vi "Core Action.vi"(8 "error in (no error)":errorcluster, 10 "SECS-II Class":refnum<class "SECS-II Class.lvclass">, 11 "30-Host Requests Equipment to Set Time in":refnum<class "30-Host Requests Equipment to Set Time.lvclass">) -> (0 "error out":errorcluster, 2 "SECS-II Class Out":refnum<class "SECS-II Class.lvclass">, 3 "30-Host Requests Equipment to Set Time out":refnum<class "30-Host Requests Equipment to Set Time.lvclass">)   [LabVIEW 2020, in "SECS Scenarios.lvlib" / "30-Host Requests Equipment to Set Time.lvclass"]
uses:
  30-Host Requests Equipment to Set Time.lvclass
  D:/Dropbox/SECS/SECS_GEM v1.1.0/Com/SECS Scenarios/Scenarios Class/Scenarios Class.lvclass
  SECS Communication/SECS-II Class/SECS-II Class.lvclass
  SECS Communication/S2 Message Class/S2 Message Class.lvclass
  D:/Dropbox/SECS/SECS_GEM v1.1.0/Com/SECS Communication/SECS-II Class/SECS-II Class.lvclass
  Scenarios Class/Reply State.ctl
  Scenarios Class/Scenarios Class.lvclass/Scenarios Class.ctl
  Scenarios Class/Write Reply State.vi
  Scenarios Class/Read HSMS Class.vi
  SECS Communication/HSMS Class/HSMS Class.lvclass
  Scenarios Class/Scenarios Class.lvclass
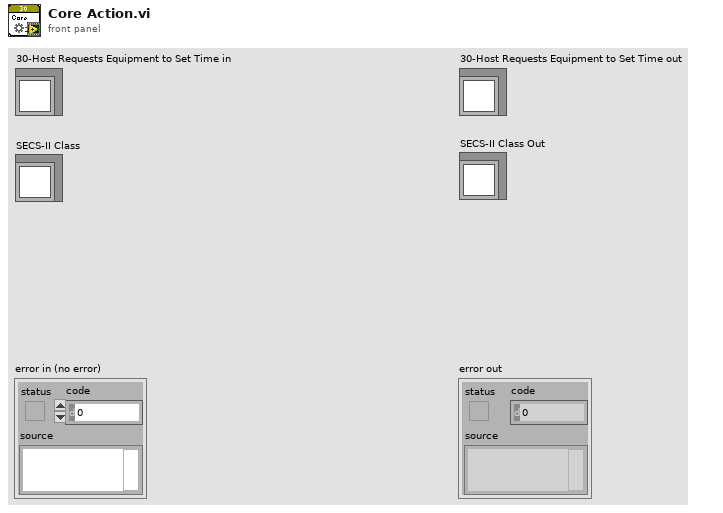
[diagram p1: front panel]
types:
  T1 = typedef "SECS Scenarios.lvlib/Scenarios Class.lvclass/Reply State.ctl" = enum16{"OK", "Illegal Data", "Unknown Stream", "Unknown Function", "Off-Line", "T3 Timeout", "Inner-Timeout"}
  T2 = typedef "SECS Communication.lvlib/S2 Message Class.lvclass/S2F32.ctl" = enum16{"ok", "not done"}
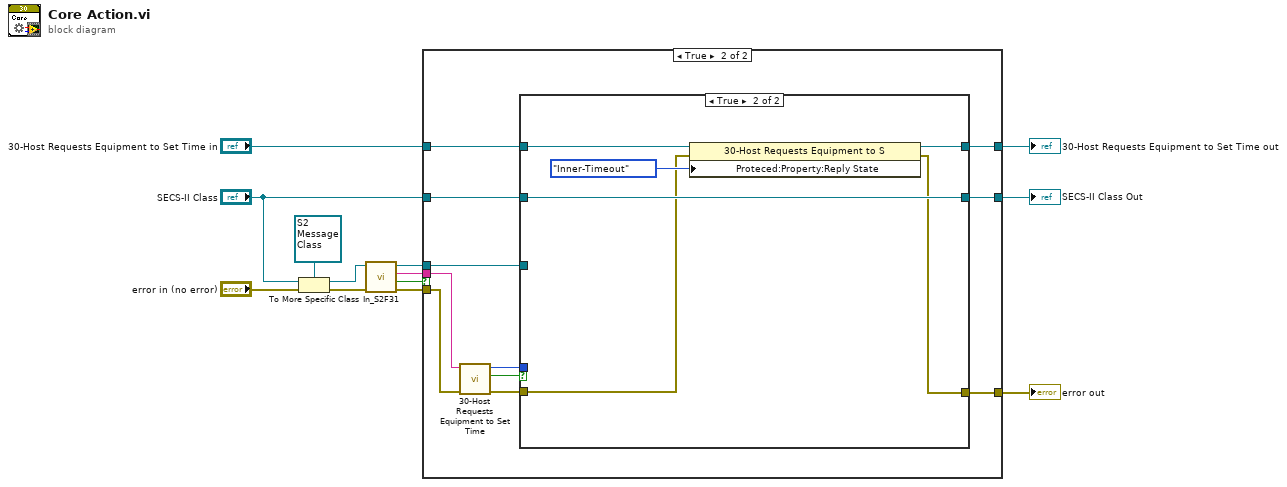
[diagram p0: block diagram]
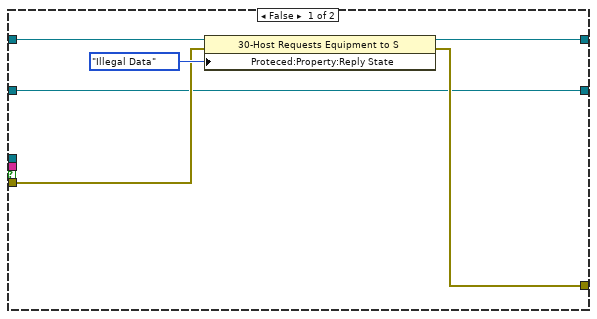
[diagram p2: hidden frame]
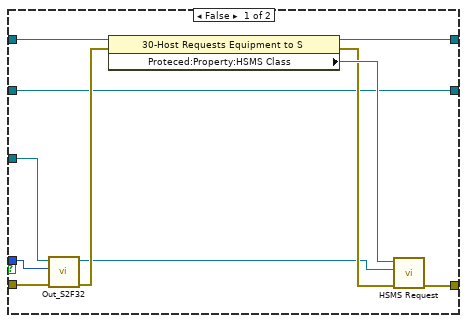
[diagram p3: hidden frame]
diagram:
  n1 = To More Specific Class(target class=refnum<class "S2 Message Class.lvclass"> refnum ("SECS Communication.lvlib:S2 Message Class.lvclass"), reference="SECS-II Class", error in="error in (no error)") -> (specific class reference=w12:refnum<class "S2 Message Class.lvclass">, error out=w13:errorcluster)
  n2 = call "In_S2F31.vi"("error in (no error)"=w13, "S2 Message Class in"=w12) -> ("error out"=w11:errorcluster, "OK?"=w1:bool, "Time"=w9:string, "S2 Message Class out"=w10:refnum<class "S2 Message Class.lvclass">)  [unwired: 6 in]
  n3 = case shown="True" w1 {
    tunnel: w11 -> [w16 w30]
    tunnel: w10 -> [_ w29]
    tunnel: w9 -> [_ w26]
    tunnel: "30-Host Requests Equipment to Set Time in" -> [w19 w24]
    tunnel: [w15 w23] -> w5
    tunnel: [w18 w22] -> w4
    tunnel: "SECS-II Class" -> [w14 w21]
    tunnel: [w14 w20] -> w2
    frame False {
      n4 = property class="30-Host Requests Equipment to S"(reference=w19, error in=w16, "Proteced:Property:Reply State"=Reply_State."Illegal Data" ("Reply State")) -> (reference out=w18:refnum<class "30-Host Requests Equipment to Set Time.lvclass">, error out=w15:errorcluster)
    }
    frame True {
      n5 = call "30-Host Requests Equipment to Set Time.vi"("error in (no error)"=w30, "Time"=w26) -> ("error out"=w28:errorcluster, "Timeout?"=w27:bool, "S2F32"=w25:T2)  [unwired: 7 in]
      n6 = case shown="True" w27 {
        tunnel: w24 -> [w41 w45]
        tunnel: w29 -> [w37 _]
        tunnel: [w32 w42] -> w23
        tunnel: [w38 w43] -> w22
        tunnel: w28 -> [w34 w44]
        tunnel: w25 -> [w33 _]
        tunnel: w21 -> [w31 w47]
        tunnel: [w31 w47] -> w20
        frame False {
          n7 = call "Out_S2F32.vi"("error in (no error)"=w34, "S2F32"=w33, "S2 Message Class in"=w37) -> ("error out"=w36:errorcluster, "S2 Message Class out"=w35:refnum<class "S2 Message Class.lvclass">)  [unwired: 7 in]
          n8 = property class="30-Host Requests Equipment to S"(reference=w41, error in=w36) -> (reference out=w38:refnum<class "30-Host Requests Equipment to Set Time.lvclass">, error out=w39:errorcluster, "Proteced:Property:HSMS Class"=w40:refnum<class "HSMS Class.lvclass">)
          n9 = call "HSMS Request.vi"("error in (no error)"=w39, "SECS-II Class In"=w35, "HSMS Class in"=w40) -> ("error out"=w32:errorcluster)  [unwired: 7 in, 1 out]
        }
        frame True {
          n10 = property class="30-Host Requests Equipment to S"(reference=w45, error in=w44, "Proteced:Property:Reply State"=Reply_State."Inner-Timeout" ("Reply State")) -> (reference out=w43:refnum<class "30-Host Requests Equipment to Set Time.lvclass">, error out=w42:errorcluster)
        }
      }
    }
  }
  "error out" <- w5
  "30-Host Requests Equipment to Set Time out" <- w4
  "SECS-II Class Out" <- w2
